vi "Mecanum_Begin.vi"(11 "Brake?":bool) -> ()   [LabVIEW 2012]
uses:
  <vilib>/Rock Robotics/WPI/CAN/Jaguar/SubVIs/WPI_CANJaguar_SpeedReference.ctl
  <vilib>/Rock Robotics/WPI/CAN/Jaguar/SubVIs/WPI_CANJaguar_BrakeCoastMode.ctl
  <vilib>/Rock Robotics/WPI/CAN/Jaguar/SubVIs/WPI_CANJaguar_ControlMode.ctl
  <vilib>/Rock Robotics/WPI/MotorControl/WPI_MotorControlOpenCANJaguar.vi
panel:
  out "Succeeded?":bool
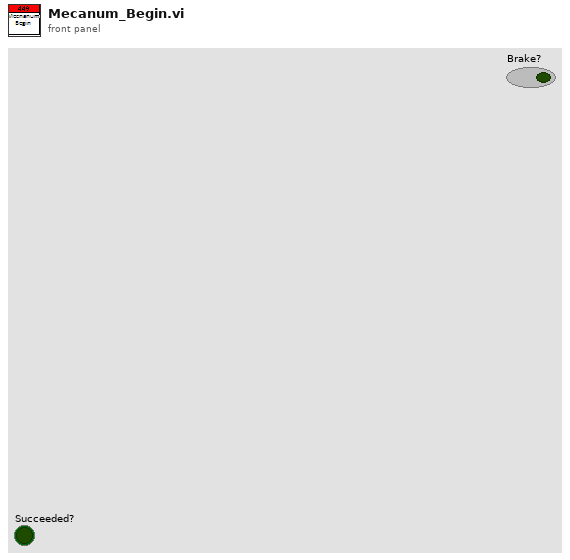
[diagram p1: front panel]
types:
  T1 = typedef "WPI_CANJaguar_BrakeCoastMode.ctl" = enum8{"Jumper", "Brake", "Coast"}
  T2 = typedef "WPI_CANJaguar_SpeedReference.ctl" = u8
  T3 = typedef "WPI_CANJaguar_ControlMode.ctl" = enum8{"Percent VBus", "Current", "Speed", "Position", "Voltage"}
  T4 = typedef "WPI_MotorControlDeviceRef.ctl" = cluster{"DeviceStatus":errorcluster, "Type":enum16{"PWM", "CAN"}, "PWM":cluster{"Digital Module":T5, "PWM Channel":T6, "DeadBand":T7}, "CAN":cluster{"Device Number":u8, "Control Mode":T3, "Semaphore":T8, "Max Vout":dbl}, "Invert":bool, "TransformRef":T9, "InvTransformRef":T9}
  T5 = typedef "FPGA_TypedefDigitalModule.ctl" = enum16{"Digital Module 1", "Digital Module 2"}
  T6 = typedef "FPGA_DIOPWMChannel.ctl" = enum8{"PWM 1", "PWM 2", "PWM 3", "PWM 4", "PWM 5", "PWM 6", "PWM 7", "PWM 8", "PWM 9", "PWM 10", "Invalid"}
  T7 = typedef "WPI_PWMDeadband.ctl" = cluster{"Name":string, "maxPositivePwm":i32, "minPositivePwm":i32, "centerPwm":i32, "maxNegativePwm":i32, "minNegativePwm":i32, "angularRange":u16}
  T8 = typedef "Semaphore RefNum" = refnum<k1>
  T9 = typedef "WPI_PWMTransform_ConPane.ctl" = refnum<vi>
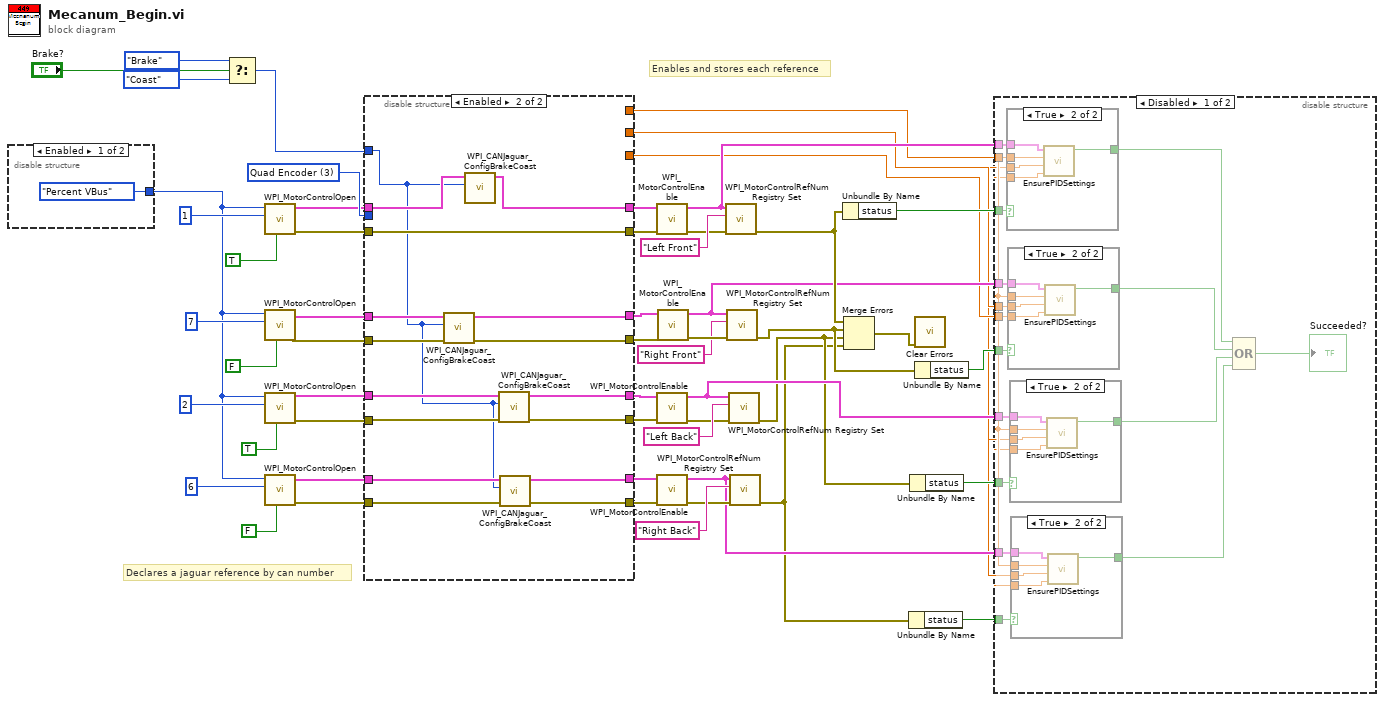
[diagram p0: block diagram]
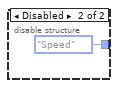
[diagram p2: hidden frame]
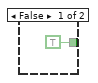
[diagram p3: hidden frame]
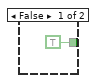
[diagram p4: hidden frame]
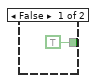
[diagram p5: hidden frame]
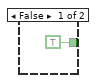
[diagram p6: hidden frame]
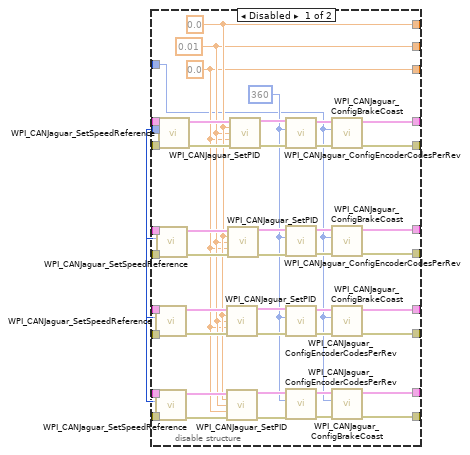
[diagram p8: hidden frame]
diagram:
  w46 = T2 3 items=["Encoder"=0, "Inv Encoder"=2, "Quad Encoder"=3, "None"=255] ("Speed Reference")
  # "Enables and stores each reference"
  # "Declares a jaguar reference by can number"
  n1 = disable-structure shown="Enabled" {
    disable-tunnel: [WPI_CANJaguar_ControlMode."Percent VBus" ("Control Mode") WPI_CANJaguar_ControlMode."Speed" ("Control Mode")] -> w44
    frame Enabled {
    }
    frame Disabled {
    }
  }
  n2 = Select(t=WPI_CANJaguar_BrakeCoastMode."Brake" ("Brake / Coast Mode"), s="Brake?", f=WPI_CANJaguar_BrakeCoastMode."Coast") -> (s? t:f=w4:T1)
  n3 = call-poly <vilib>:"WPI_MotorControlOpen.vi"("Invert"=TRUE, "Device Number"=u8 1, "Control Mode"=w44) -> ("error out"=w42:errorcluster, "MotorControlDeviceRef"=w43:T4)  [unwired: 3 in, 4 out]
  n4 = call-poly <vilib>:"WPI_MotorControlOpen.vi"("Invert"=FALSE, "Device Number"=u8 7, "Control Mode"=w44) -> ("error out"=w24:errorcluster, "MotorControlDeviceRef"=w25:T4)  [unwired: 3 in, 4 out]
  n5 = call-poly <vilib>:"WPI_MotorControlOpen.vi"("Invert"=TRUE, "Device Number"=u8 2, "Control Mode"=w44) -> ("error out"=w48:errorcluster, "MotorControlDeviceRef"=w47:T4)  [unwired: 3 in, 4 out]
  n6 = call-poly <vilib>:"WPI_MotorControlOpen.vi"("Invert"=FALSE, "Device Number"=u8 6, "Control Mode"=w44) -> ("error out"=w49:errorcluster, "MotorControlDeviceRef"=w50:T4)  [unwired: 3 in, 4 out]
  n7 = disable-structure shown="Enabled" {
    disable-tunnel: w50 -> [w102 w110]
    disable-tunnel: w49 -> [w101 w109]
    disable-tunnel: w48 -> [w100 w111]
    disable-tunnel: w47 -> [w99 w112]
    disable-tunnel: w46 -> [w98 _]
    disable-tunnel: w43 -> [w97 w108]
    disable-tunnel: w42 -> [w96 w115]
    disable-tunnel: [w89 w107] -> w38
    disable-tunnel: [w88 w115] -> w37
    disable-tunnel: [w81 w111] -> w34
    disable-tunnel: [w80 w105] -> w33
    disable-tunnel: [w73 w104] -> w30
    disable-tunnel: [w72 w109] -> w29
    disable-tunnel: w25 -> [w69 w114]
    disable-tunnel: w24 -> [w68 w113]
    disable-tunnel: [w63 w113] -> w23
    disable-tunnel: [w62 w106] -> w22
    disable-tunnel: [w61 _] -> w15
    disable-tunnel: [w60 _] -> w14
    disable-tunnel: [w59 _] -> w13
    disable-tunnel: w4 -> [w57 w103]
    frame Disabled {
      w58 = u16 360 ("Encoder Codes Per Rev")
      w59 = 0.0 ("P")
      w60 = 0.01 ("P")
      w61 = 0.0 ("P")
      n8 = call <vilib>:"WPI_CANJaguar_SetSpeedReference.vi"("error in (no error)"=w100, "Speed Reference"=w98, "CAN Jaguar Ref"=w99) -> ("error out"=w87:errorcluster, "CAN Jaguar Ref Out"=w86:T4)  [unwired: 7 in]
      n9 = call <vilib>:"WPI_CANJaguar_SetSpeedReference.vi"("error in (no error)"=w101, "Speed Reference"=w98, "CAN Jaguar Ref"=w102) -> ("error out"=w79:errorcluster, "CAN Jaguar Ref Out"=w78:T4)  [unwired: 7 in]
      n10 = call <vilib>:"WPI_CANJaguar_SetSpeedReference.vi"("error in (no error)"=w68, "Speed Reference"=w98, "CAN Jaguar Ref"=w69) -> ("error out"=w71:errorcluster, "CAN Jaguar Ref Out"=w70:T4)  [unwired: 7 in]
      n11 = call <vilib>:"WPI_CANJaguar_SetSpeedReference.vi"("error in (no error)"=w96, "Speed Reference"=w98, "CAN Jaguar Ref"=w97) -> ("error out"=w94:errorcluster, "CAN Jaguar Ref Out"=w95:T4)  [unwired: 7 in]
      n12 = call <vilib>:"WPI_CANJaguar_SetPID.vi"("CAN Jaguar Ref"=w86, "P"=w61, "I"=w60, "D"=w59, "error in (no error)"=w87) -> ("CAN Jaguar Ref Out"=w82:T4, "error out"=w83:errorcluster)  [unwired: 9 in]
      n13 = call <vilib>:"WPI_CANJaguar_SetPID.vi"("CAN Jaguar Ref"=w78, "P"=w61, "I"=w60, "D"=w59, "error in (no error)"=w79) -> ("CAN Jaguar Ref Out"=w74:T4, "error out"=w75:errorcluster)  [unwired: 9 in]
      n14 = call <vilib>:"WPI_CANJaguar_SetPID.vi"("CAN Jaguar Ref"=w70, "P"=w61, "I"=w60, "D"=w59, "error in (no error)"=w71) -> ("CAN Jaguar Ref Out"=w64:T4, "error out"=w65:errorcluster)  [unwired: 9 in]
      n15 = call <vilib>:"WPI_CANJaguar_SetPID.vi"("CAN Jaguar Ref"=w95, "P"=w61, "I"=w60, "D"=w59, "error in (no error)"=w94) -> ("CAN Jaguar Ref Out"=w90:T4, "error out"=w91:errorcluster)  [unwired: 9 in]
      n16 = call <vilib>:"WPI_CANJaguar_ConfigEncoderCodesPerRev.vi"("error in (no error)"=w91, "Encoder Codes Per Rev"=w58, "CAN Jaguar Ref"=w90) -> ("error out"=w92:errorcluster, "CAN Jaguar Ref Out"=w93:T4)  [unwired: 7 in]
      n17 = call <vilib>:"WPI_CANJaguar_ConfigEncoderCodesPerRev.vi"("error in (no error)"=w65, "Encoder Codes Per Rev"=w58, "CAN Jaguar Ref"=w64) -> ("error out"=w66:errorcluster, "CAN Jaguar Ref Out"=w67:T4)  [unwired: 7 in]
      n18 = call <vilib>:"WPI_CANJaguar_ConfigEncoderCodesPerRev.vi"("error in (no error)"=w83, "Encoder Codes Per Rev"=w58, "CAN Jaguar Ref"=w82) -> ("error out"=w85:errorcluster, "CAN Jaguar Ref Out"=w84:T4)  [unwired: 7 in]
      n19 = call <vilib>:"WPI_CANJaguar_ConfigEncoderCodesPerRev.vi"("error in (no error)"=w75, "Encoder Codes Per Rev"=w58, "CAN Jaguar Ref"=w74) -> ("error out"=w76:errorcluster, "CAN Jaguar Ref Out"=w77:T4)  [unwired: 7 in]
      n20 = call <vilib>:"WPI_CANJaguar_ConfigBrakeCoast.vi"("error in (no error)"=w92, "Brake / Coast Mode"=w57, "CAN Jaguar Ref"=w93) -> ("error out"=w88:errorcluster, "CAN Jaguar Ref Out"=w89:T4)  [unwired: 7 in]
      n21 = call <vilib>:"WPI_CANJaguar_ConfigBrakeCoast.vi"("error in (no error)"=w66, "Brake / Coast Mode"=w57, "CAN Jaguar Ref"=w67) -> ("error out"=w63:errorcluster, "CAN Jaguar Ref Out"=w62:T4)  [unwired: 7 in]
      n22 = call <vilib>:"WPI_CANJaguar_ConfigBrakeCoast.vi"("error in (no error)"=w85, "Brake / Coast Mode"=w57, "CAN Jaguar Ref"=w84) -> ("error out"=w81:errorcluster, "CAN Jaguar Ref Out"=w80:T4)  [unwired: 7 in]
      n23 = call <vilib>:"WPI_CANJaguar_ConfigBrakeCoast.vi"("error in (no error)"=w76, "Brake / Coast Mode"=w57, "CAN Jaguar Ref"=w77) -> ("error out"=w72:errorcluster, "CAN Jaguar Ref Out"=w73:T4)  [unwired: 7 in]
    }
    frame Enabled {
      n24 = call <vilib>:"WPI_CANJaguar_ConfigBrakeCoast.vi"("Brake / Coast Mode"=w103, "CAN Jaguar Ref"=w114) -> ("CAN Jaguar Ref Out"=w106:T4)  [unwired: 8 in, 1 out]
      n25 = call <vilib>:"WPI_CANJaguar_ConfigBrakeCoast.vi"("Brake / Coast Mode"=w103, "CAN Jaguar Ref"=w108) -> ("CAN Jaguar Ref Out"=w107:T4)  [unwired: 8 in, 1 out]
      n26 = call <vilib>:"WPI_CANJaguar_ConfigBrakeCoast.vi"("Brake / Coast Mode"=w103, "CAN Jaguar Ref"=w112) -> ("CAN Jaguar Ref Out"=w105:T4)  [unwired: 8 in, 1 out]
      n27 = call <vilib>:"WPI_CANJaguar_ConfigBrakeCoast.vi"("Brake / Coast Mode"=w103, "CAN Jaguar Ref"=w110) -> ("CAN Jaguar Ref Out"=w104:T4)  [unwired: 8 in, 1 out]
    }
  }
  n28 = call <vilib>:"WPI_MotorControlEnable.vi"("error in (no error)"=w37, "CAN Jaguar Ref"=w38) -> ("error out"=w39:errorcluster, "CAN Jaguar Ref Out"=w20:T4)  [unwired: 1 in, 7 out]
  n29 = call <vilib>:"WPI_MotorControlEnable.vi"("error in (no error)"=w34, "CAN Jaguar Ref"=w33) -> ("error out"=w35:errorcluster, "CAN Jaguar Ref Out"=w17:T4)  [unwired: 1 in, 7 out]
  n30 = call <vilib>:"WPI_MotorControlEnable.vi"("error in (no error)"=w29, "CAN Jaguar Ref"=w30) -> ("error out"=w31:errorcluster, "CAN Jaguar Ref Out"=w16:T4)  [unwired: 1 in, 7 out]
  n31 = call <vilib>:"WPI_MotorControlEnable.vi"("error in (no error)"=w23, "CAN Jaguar Ref"=w22) -> ("error out"=w26:errorcluster, "CAN Jaguar Ref Out"=w18:T4)  [unwired: 1 in, 7 out]
  n32 = call <vilib>:"WPI_MotorControlRefNum Registry Set.vi"("error in (no error)"=w39, "refnum name"="Left Front", "MotorControlDevRef"=w20) -> ("error out"=w21:errorcluster)  [unwired: 8 out]
  n33 = call <vilib>:"WPI_MotorControlRefNum Registry Set.vi"("error in (no error)"=w26, "refnum name"="Right Front", "MotorControlDevRef"=w18) -> ("error out"=w12:errorcluster)  [unwired: 8 out]
  n34 = call <vilib>:"WPI_MotorControlRefNum Registry Set.vi"("error in (no error)"=w35, "refnum name"="Left Back", "MotorControlDevRef"=w17) -> ("error out"=w10:errorcluster)  [unwired: 8 out]
  n35 = call <vilib>:"WPI_MotorControlRefNum Registry Set.vi"("error in (no error)"=w31, "refnum name"="Right Back", "MotorControlDevRef"=w16) -> ("error out"=w8:errorcluster)  [unwired: 8 out]
  n36 = Unbundle By Name(w21) -> ("status"=w19:bool)
  n37 = Merge Errors(w21, w12, w10, w8) -> (w1:errorcluster)
  n38 = Unbundle By Name(w8) -> ("status"=w7:bool)
  n39 = Unbundle By Name(w10) -> ("status"=w9:bool)
  n40 = call <vilib>:"Clear Errors.vi"("error in (no error)"=w1) -> ()  [unwired: 6 in, 1 out]
  n41 = Unbundle By Name(w12) -> ("status"=w11:bool)
  n42 = disable-structure shown="Disabled" {
    disable-tunnel: w20 -> [w131 _]
    disable-tunnel: w19 -> [w130 _]
    disable-tunnel: w18 -> [w129 _]
    disable-tunnel: w17 -> [w128 _]
    disable-tunnel: w16 -> [w127 _]
    disable-tunnel: w15 -> [w126 _]
    disable-tunnel: w14 -> [w125 _]
    disable-tunnel: w13 -> [w124 _]
    disable-tunnel: w11 -> [w123 _]
    disable-tunnel: w9 -> [w122 _]
    disable-tunnel: w7 -> [w121 _]
    frame Disabled {
      n43 = case shown="True" w130 {
        tunnel: w131 -> [_ w155]
        tunnel: w126 -> [_ w154]
        tunnel: w125 -> [_ w153]
        tunnel: w124 -> [_ w152]
        tunnel: [TRUE ("Succeeded?") w151] -> w120
        frame False {
        }
        frame True {
          n44 = call "EnsurePIDSettings.vi"("D"=w152, "I"=w153, "P"=w154, "CAN Jaguar Ref"=w155) -> ("Succeeded?"=w151:bool)  [unwired: 7 in]
        }
      }
      n45 = case shown="True" w123 {
        tunnel: w129 -> [_ w149]
        tunnel: w126 -> [_ w148]
        tunnel: w125 -> [_ w147]
        tunnel: w124 -> [_ w146]
        tunnel: [TRUE ("Succeeded?") w145] -> w119
        frame False {
        }
        frame True {
          n46 = call "EnsurePIDSettings.vi"("D"=w146, "I"=w147, "P"=w148, "CAN Jaguar Ref"=w149) -> ("Succeeded?"=w145:bool)  [unwired: 7 in]
        }
      }
      n47 = case shown="True" w122 {
        tunnel: w128 -> [_ w143]
        tunnel: w126 -> [_ w142]
        tunnel: w125 -> [_ w141]
        tunnel: w124 -> [_ w140]
        tunnel: [TRUE ("Succeeded?") w139] -> w117
        frame False {
        }
        frame True {
          n48 = call "EnsurePIDSettings.vi"("D"=w140, "I"=w141, "P"=w142, "CAN Jaguar Ref"=w143) -> ("Succeeded?"=w139:bool)  [unwired: 7 in]
        }
      }
      n49 = case shown="True" w121 {
        tunnel: w127 -> [_ w137]
        tunnel: w126 -> [_ w136]
        tunnel: w125 -> [_ w135]
        tunnel: w124 -> [_ w134]
        tunnel: [TRUE ("Succeeded?") w133] -> w118
        frame False {
        }
        frame True {
          n50 = call "EnsurePIDSettings.vi"("D"=w134, "I"=w135, "P"=w136, "CAN Jaguar Ref"=w137) -> ("Succeeded?"=w133:bool)  [unwired: 7 in]
        }
      }
      n51 = Compound Arithmetic op=OR(w120, w119, w117, w118) -> (→"Succeeded?":bool)
    }
    frame Enabled {
    }
  }
